vi "Y Limiter.vi"(5 "reinitialize? (F)":bool, 7 "X1(SetState)":T1(ring)=enum."max", 9 "Y param":T3={"output high"=100.0, "alr value"=0.0, "output low"=0.0, "output time (t)"=1.0} {"output time (t)" format="%.2f"; "output low" format="%.3f"; "alr value" format="%.3f"; "output high" format="%.3f"}, 10 "Y (NaN)":dbl=nan, 11 "Y_Set":dbl) -> (1 "End":bool, 2 "SpLim_State":T2=enum."increase", 3 "output":dbl format="%.2f")   [LabVIEW 2019, in "control.lvlib"]
uses:
  control.lvlib
  ctl/control param simple.ctl
  ctl/Y_Lim_State.ctl
  PID Timing Estimation.vi
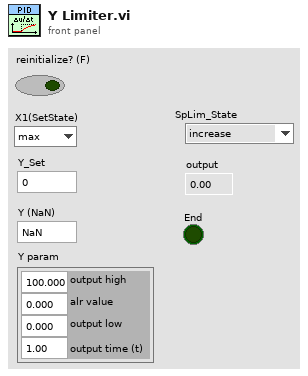
[diagram p1: front panel]
types:
  T1 = enum8{"alarm", "min", "stop", "hand", "auto", "max"}
  T2 = typedef "Y_Lim_State.ctl" = enum8{"initialization", "alarm", "stop", "decrease", "increase"}
  T3 = typedef "control.lvlib/control param simple.ctl" = cluster{"output high":dbl, "alr value":dbl, "output low":dbl, "output time (t)":dbl}
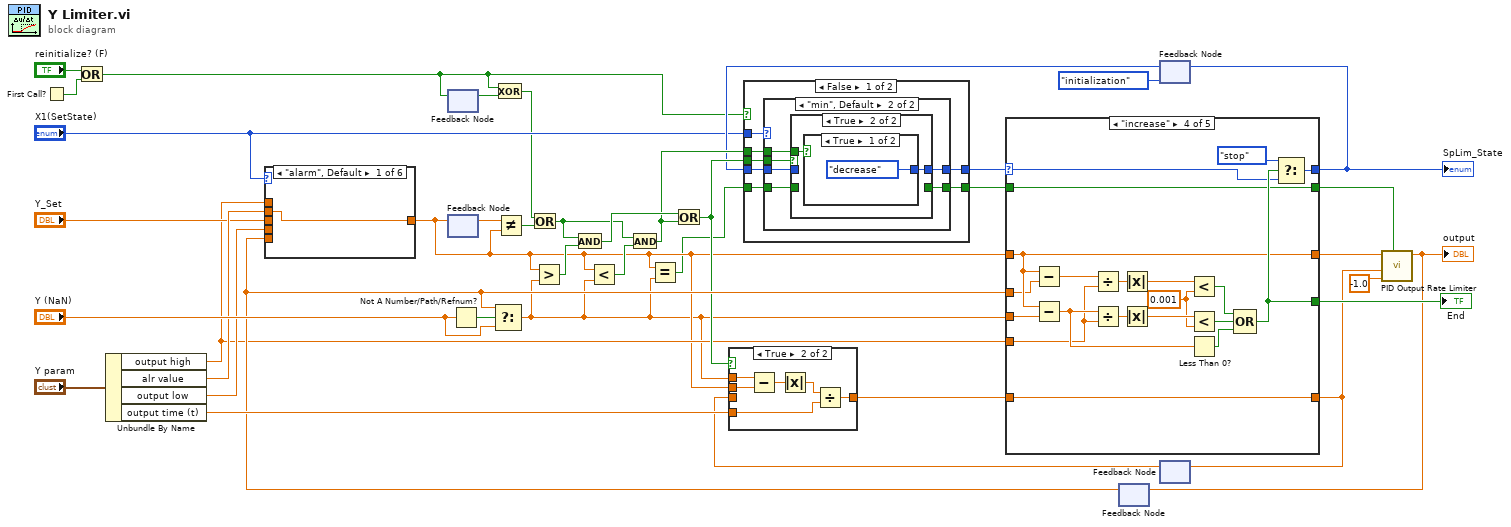
[diagram p0: block diagram]
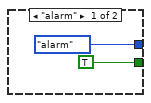
[diagram p7: hidden frame]
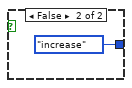
[diagram p9: hidden frame]
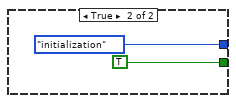
[diagram p10: hidden frame]
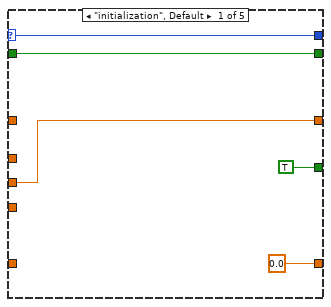
[diagram p12: hidden frame]
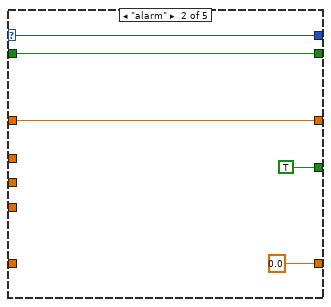
[diagram p13: hidden frame]
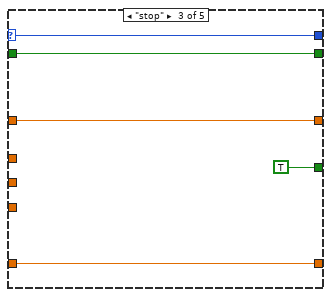
[diagram p14: hidden frame]
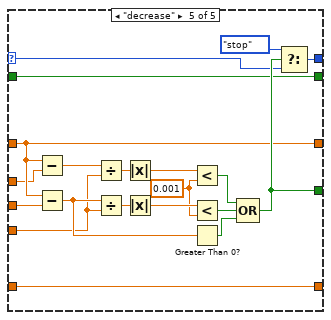
[diagram p15: hidden frame]
diagram:
  n1 = First Call?() -> (First Call?: T/F=w19:bool)
  n2 = Or(x="reinitialize? (F)", y=w19) -> (x .or. y?=w6:bool)
  n3 = Unbundle By Name("Y param") -> ("output high"=w8:dbl, "alr value"=w18:dbl, "output low"=w17:dbl, "output time (t)"=w35:dbl)
  n4 = feedback #1() -> (w7:bool)  [unwired: 1 in]
  n5 = feedback-in #1(w6) -> ()
  n6 = feedback #2() -> (w30:dbl)  [unwired: 1 in]
  n7 = Not A Number/Path/Refnum?(number/path/refnum="Y (NaN)") -> (NaN/Path/Refnum?=w32:bool)
  n8 = Exclusive Or(1:w7, 2:w6) -> (0:w4:bool)
  n9 = feedback #3() -> (w15:dbl)  [unwired: 1 in]
  n10 = case shown="\"alarm\", Default" "X1(SetState)" {
    tunnel: w8 -> [_ _ _ _ _ w45]
    tunnel: w18 -> [w40 _ _ _ _ _]
    tunnel: w17 -> [_ w41 _ _ _ _]
    tunnel: "Y_Set" -> [_ _ _ w43 w44 _]
    tunnel: [w40 w41 w42 w43 w44 w45] -> w3
    tunnel: w15 -> [_ _ w42 _ _ _]
    frame "alarm", Default {
    }
    frame "min" {
    }
    frame "stop" {
    }
    frame "hand" {
    }
    frame "auto" {
    }
    frame "max" {
    }
  }
  n11 = feedback-in #2(w3) -> ()
  n12 = Select(t=w15, s=w32, f="Y (NaN)") -> (s? t:f=w2:dbl)
  n13 = Not Equal?(x=w30, y=w3) -> (x != y?=w27:bool)
  n14 = Or(x=w4, y=w27) -> (x .or. y?=w5:bool)
  n15 = Greater?(x=w3, y=w2) -> (0:w29:bool)
  n16 = And(x=w5, y=w29) -> (x .and. y?=w28:bool)
  n17 = Less?(x=w3, y=w2) -> (x < y?=w26:bool)
  n18 = And(x=w5, y=w26) -> (x .and. y?=w13:bool)
  n19 = Equal?(x=w3, y=w2) -> (x = y?=w1:bool)
  n20 = Or(x=w28, y=w13) -> (x .or. y?=w14:bool)
  n21 = feedback #4(Y_Lim_State."initialization" ("SpLim_State")) -> (w12:T2)
  n22 = case shown="False" w6 {
    tunnel: [w51 Y_Lim_State."initialization" ("SpLim_State")] -> w11
    tunnel: [w47 TRUE] -> w9
    tunnel: w14 -> [w52 _]
    tunnel: w13 -> [w50 _]
    tunnel: w12 -> [w49 _]
    tunnel: "X1(SetState)" -> [w48 _]
    tunnel: w1 -> [w46 _]
    frame False {
      n23 = case shown="\"min\", Default" w48 {
        tunnel: w52 -> [_ w60]
        tunnel: [Y_Lim_State."alarm" ("SpLim_State") w59] -> w51
        tunnel: w50 -> [_ w58]
        tunnel: w49 -> [_ w57]
        tunnel: [TRUE w56] -> w47
        tunnel: w46 -> [_ w55]
        frame "alarm" {
        }
        frame "min", Default {
          n24 = case shown="True" w60 {
            tunnel: [w62 w64] -> w59
            tunnel: w58 -> [_ w63]
            tunnel: w57 -> [w62 _]
            tunnel: [w61 _] -> w56
            tunnel: w55 -> [w61 _]
            frame False {
            }
            frame True {
              n25 = case shown="True" w63 {
                tunnel: [Y_Lim_State."decrease" ("SpLim_State") Y_Lim_State."increase" ("SpLim_State")] -> w64
                frame True {
                }
                frame False {
                }
              }
            }
          }
        }
      }
    }
    frame True {
    }
  }
  n26 = feedback #5() -> (w21:dbl)  [unwired: 1 in]
  n27 = case shown="True" w14 {
    tunnel: w2 -> [_ w70]
    tunnel: w3 -> [_ w71]
    tunnel: w21 -> [w69 _]
    tunnel: [w69 w73] -> w33
    tunnel: w35 -> [_ w72]
    frame False {
    }
    frame True {
      n28 = Subtract(x=w70, y=w71) -> (x-y=w74:dbl)
      n29 = Absolute Value(x=w74) -> (abs(x)=w75:dbl)
      n30 = Divide(x=w75, y=w72) -> (x/y=w73:dbl)
    }
  }
  n31 = case shown="\"increase\"" w11 {
    selector: w11 -> [w76 w81 w88 w102 w122]
    tunnel: w3 -> [_ w82 w89 w100 w120]
    tunnel: w2 -> [w78 _ _ w95 w115]
    tunnel: [w78 w82 w89 w100 w120] -> w36
    tunnel: [TRUE TRUE TRUE w104 w124] -> w39
    tunnel: [0.0 0.0 w87 w106 w126] -> w22
    tunnel: [w77 w83 w86 w91 w111] -> w38
    tunnel: [w76 w81 w88 w103 w123] -> w25
    tunnel: w33 -> [_ _ w87 w106 w126]
    tunnel: w15 -> [_ _ _ w99 w119]
    tunnel: w8 -> [_ _ _ w93 w113]
    tunnel: w9 -> [w77 w83 w86 w91 w111]
    frame "initialization", Default {
    }
    frame "alarm" {
    }
    frame "stop" {
    }
    frame "increase" {
      w92 = 0.001 ("y")
      n32 = Subtract(x=w100, y=w99) -> (x-y=w96:dbl)
      n33 = Subtract(x=w100, y=w95) -> (x-y=w105:dbl)
      n34 = Divide(x=w96, y=w93) -> (x/y=w97:dbl)
      n35 = Divide(x=w105, y=w93) -> (x/y=w110:dbl)
      n36 = Absolute Value(x=w97) -> (abs(x)=w98:dbl)
      n37 = Absolute Value(x=w110) -> (abs(x)=w109:dbl)
      n38 = Less?(x=w98, y=w92) -> (x < y?=w94:bool)
      n39 = Less?(x=w109, y=w92) -> (x < y?=w108:bool)
      n40 = Less Than 0?(x=w105) -> (x < 0?=w107:bool)
      n41 = Compound Arithmetic op=OR(w94, w108, w107) -> (w104:bool)
      n42 = Select(t=Y_Lim_State."stop", s=w104, f=w102) -> (s? t:f=w103:T2)
    }
    frame "decrease" {
      w112 = 0.001 ("y")
      n43 = Subtract(x=w120, y=w119) -> (x-y=w116:dbl)
      n44 = Subtract(x=w120, y=w115) -> (x-y=w125:dbl)
      n45 = Divide(x=w116, y=w113) -> (x/y=w117:dbl)
      n46 = Divide(x=w125, y=w113) -> (x/y=w130:dbl)
      n47 = Absolute Value(x=w117) -> (abs(x)=w118:dbl)
      n48 = Absolute Value(x=w130) -> (abs(x)=w129:dbl)
      n49 = Less?(x=w118, y=w112) -> (x < y?=w114:bool)
      n50 = Less?(x=w129, y=w112) -> (x < y?=w128:bool)
      n51 = Greater Than 0?(x=w125) -> (x > 0?=w127:bool)
      n52 = Compound Arithmetic op=OR(w114, w128, w127) -> (w124:bool)
      n53 = Select(t=Y_Lim_State."stop", s=w124, f=w122) -> (s? t:f=w123:T2)
    }
  }
  "End" <- w39
  "SpLim_State" <- w25
  n54 = feedback-in #4(w25) -> ()
  n55 = feedback-in #5(w22) -> ()
  n56 = call "PID Output Rate Limiter.vi"("reinitialize? (F)"=w38, "dt (s)"=-1.0, "output rate (EGU/s)"=w22, "input (controller output)"=w36) -> ("output"=w23:dbl)  [unwired: 6 in, 1 out]
  "output" <- w23
  n57 = feedback-in #3(w23) -> ()
